vi "Main.vi"() -> ()   [LabVIEW 2015]
doc: "This template is for the Queued Message Handler design pattern.\n\nThe Event Handling Loop generates messages based on user interface actions.\n\nThe Message Handling Loop processes messages generated by the Event Handling Loop, or by other messages. The messages are string values, so new messages can be added easily to the Message Cases case structure in the Message Handling Loop. Each message cluster can also provide an optional value for Message Data, which is a variant that can be converted to whatever message-specific data is required."
uses:
  Controls & Type Defs/CurrentSong.ctl
  Controls & Type Defs/AlbumDetails.ctl
  Controls & Type Defs/UI Data.ctl
  Controls & Type Defs/AlbumArray.ctl
  Controls & Type Defs/ClickDetails.ctl
  Controls & Type Defs/SongTimerModes.ctl
  SubVIs/support/Message Queue/Enqueue Message (Single).vi
  <vilib>/Utility/error.llb/Error Cluster From Error Code.vi
  <vilib>/ErrorRing/Error Ring.xnode
  SubVIs/support/Message Queue/Message Queue.lvlib
  SubVIs/support/User Event - Stop/User Event - Stop.lvlib
panel:
  out "Album Details":T1={"Artist"="", "Album Name"="", "Songs"=-1}
  out "Current Song":T2
  in  "Pause":bool
  out "Playlist":i32(listbox)
  in  "Skip Forward":bool
  in  "Skip Back":bool
  in  "Media Stop Button":bool
  in  "Play":bool
  out "Time Remaining":dbl format="%<%M:%S>T"
  out "Song Progress":dbl(slide) scale=0.0..141.0 scale format="%<%M:%S>t"
  in  "Previous Album":bool
  in  "Next Album":bool
  out "Album Index":string
  out "Status":string
  in  "Exit":bool
  # "MP3 Player"
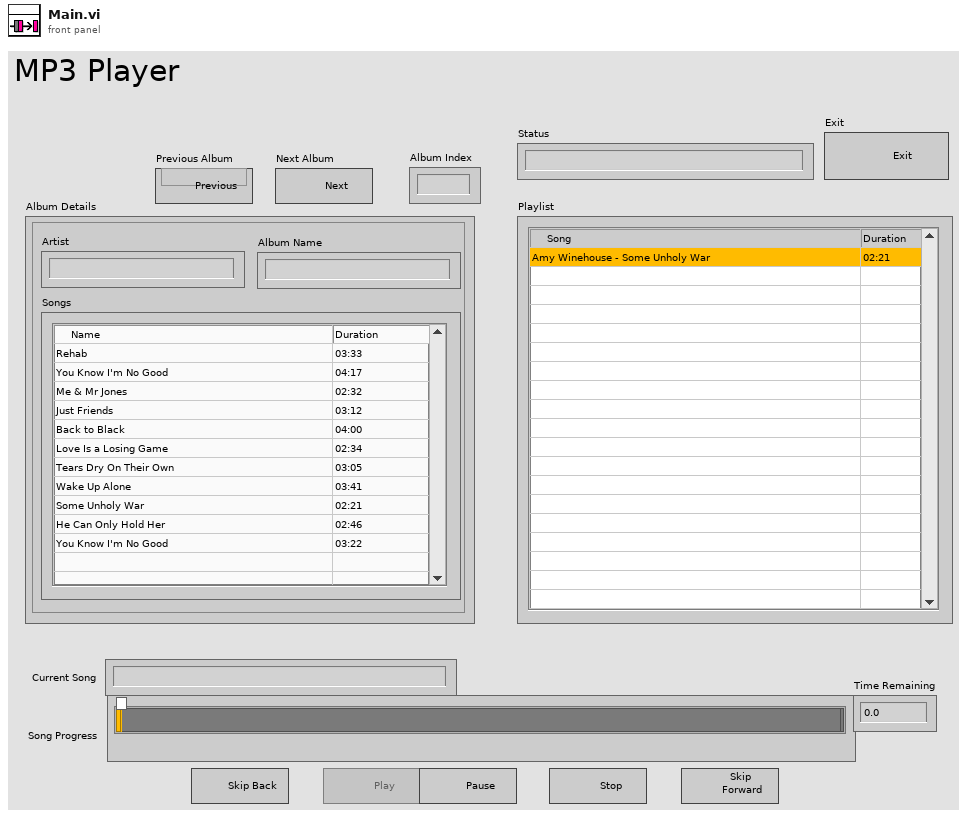
[diagram p1: front panel]
types:
  T1 = typedef "AlbumDetails.ctl" = cluster{"Artist":string, "Album Name":string, "Songs":i32}
  T2 = typedef "CurrentSong.ctl" = string
  T3 = typedef "AlbumArray.ctl" = cluster{"Artist Name":string, "Album Name":string, "Song Details":string[][]}[]
  T4 = typedef "UI Data.ctl" = cluster{"Album Index":refnum<vi>, "Album Details":refnum<vi>, "Add Button":refnum<vi>, "Remove Button":refnum<vi>, "Previous Album":refnum<vi>, "Next Album":refnum<vi>, "Song Progress":refnum<vi>, "Play":refnum<vi>, "Pause ":refnum<vi>, "Skip Forward":refnum<vi>, "Skip Back":refnum<vi>, "Media Stop Button":refnum<vi>, "Exit":refnum<vi>, "Playlist":refnum<vi>, "Current Song":refnum<vi>, "Time Remaining":refnum<vi>, "Status":refnum<vi>}
  T5 = typedef "Message Queue.lvlib/All Message Queues.ctl" = cluster{"UI":refnum<queue>, "Media":refnum<queue>}
  T6 = typedef "SongTimerModes.ctl" = enum16{"Start", "Play", "Jump"}
  T7 = typedef "ClickDetails.ctl" = cluster{"Coords":cluster{"Vertical":i32, "Horizontal":i32}, "MCLB Ref":refnum<vi>, "Button":u16}
  T8 = typedef "LVPoint32TypeDef.ctl" = cluster{"Horizontal":i32, "Vertical":i32}
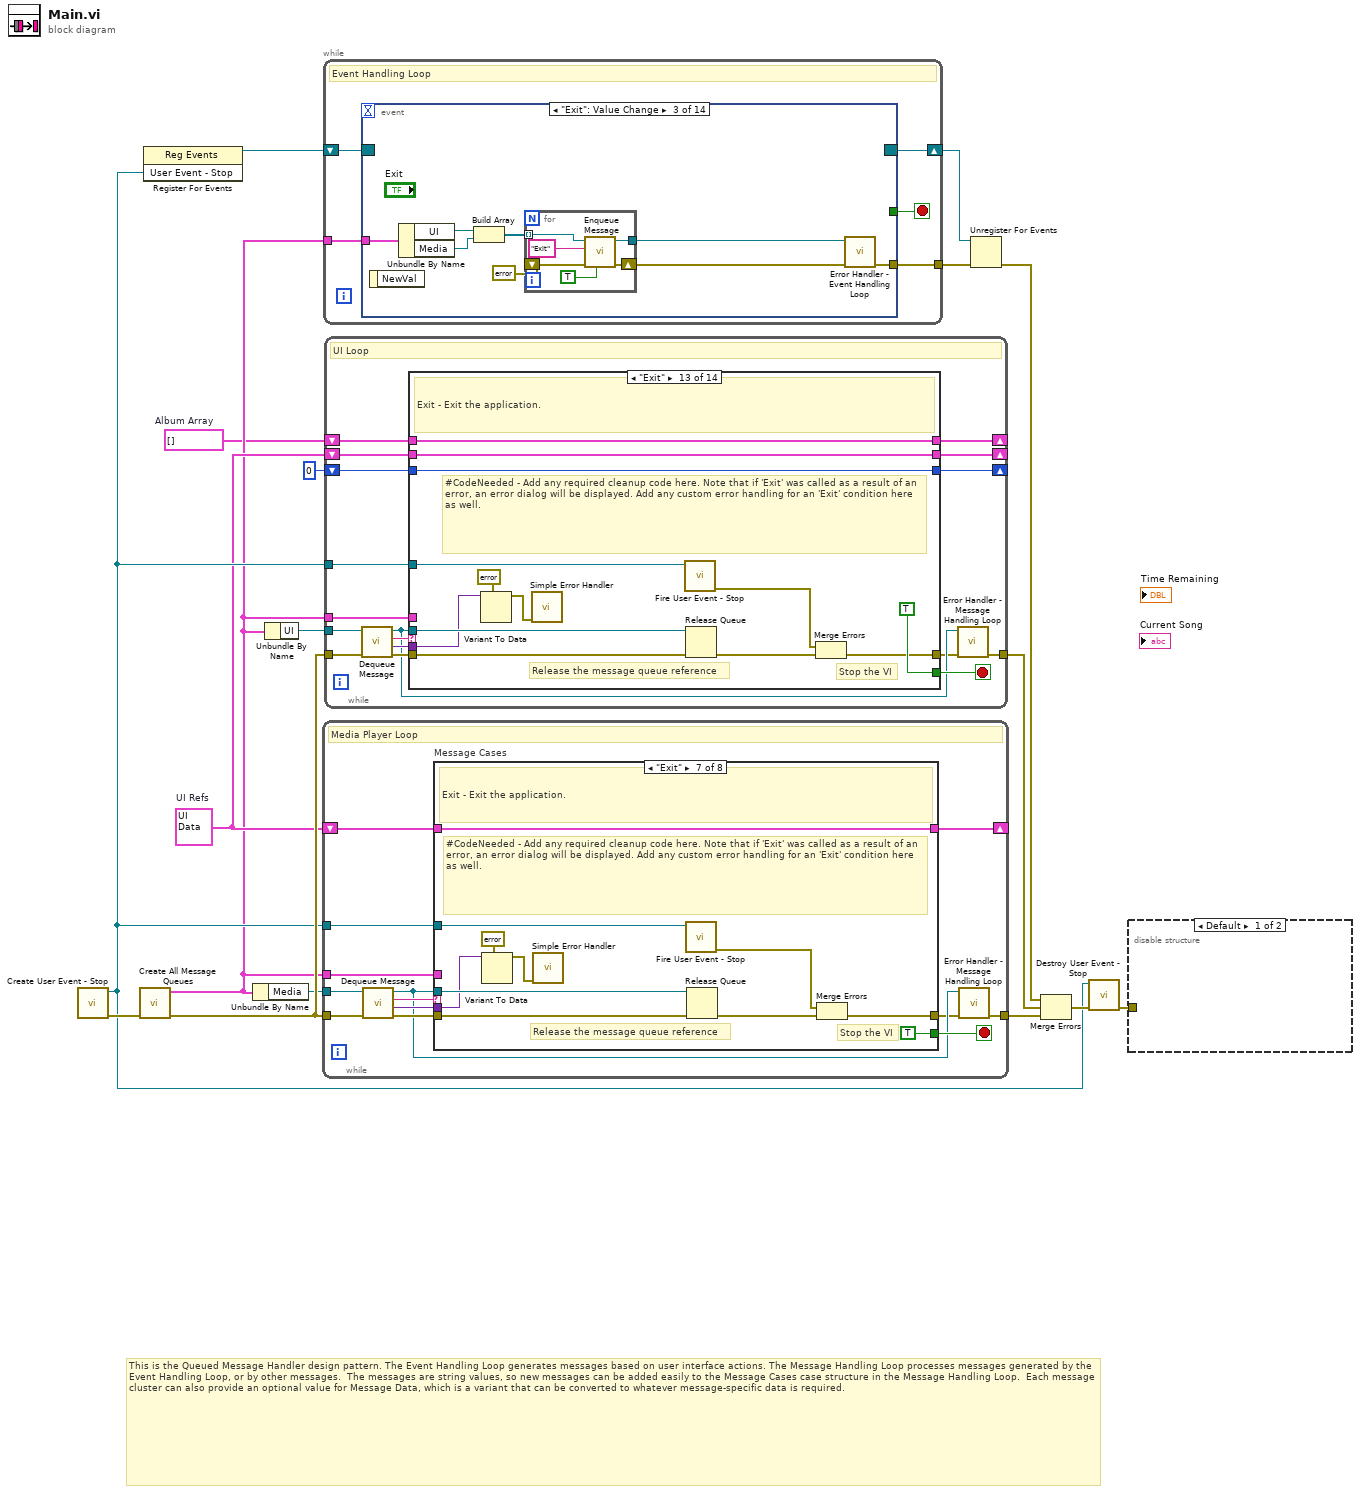
[diagram p0: block diagram]
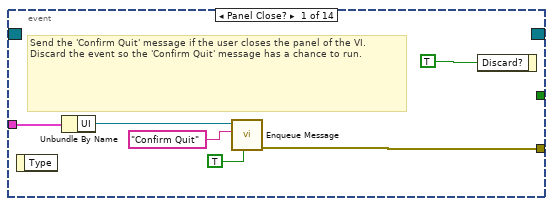
[diagram p2: hidden frame]
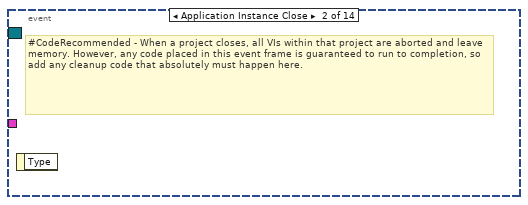
[diagram p3: hidden frame]
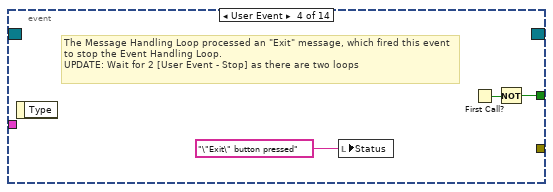
[diagram p4: hidden frame]
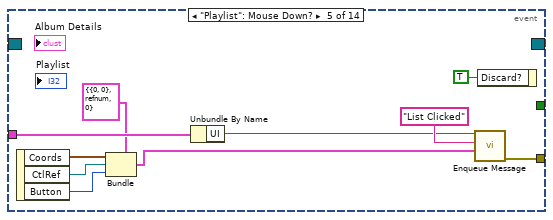
[diagram p5: hidden frame]
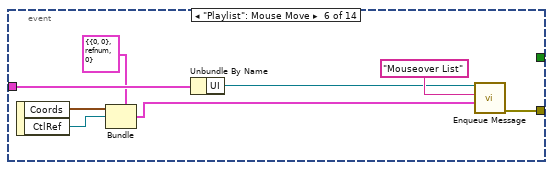
[diagram p6: hidden frame]
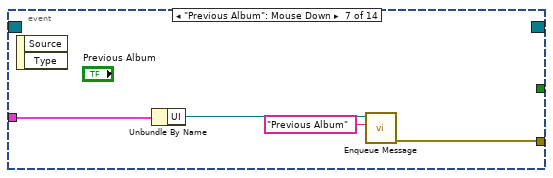
[diagram p7: hidden frame]
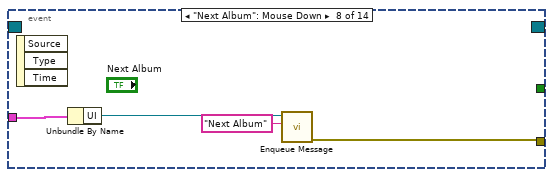
[diagram p8: hidden frame]
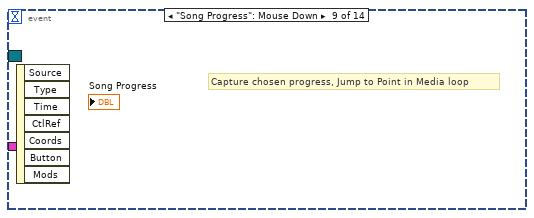
[diagram p9: hidden frame]
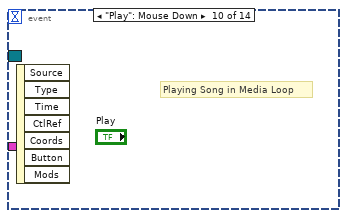
[diagram p10: hidden frame]
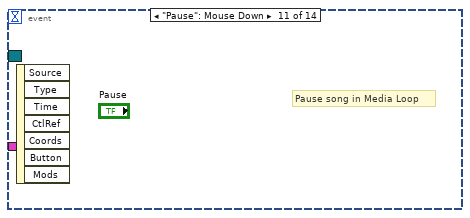
[diagram p11: hidden frame]
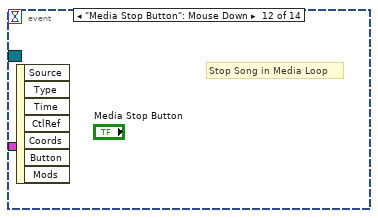
[diagram p12: hidden frame]
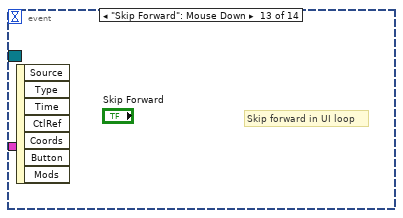
[diagram p13: hidden frame]
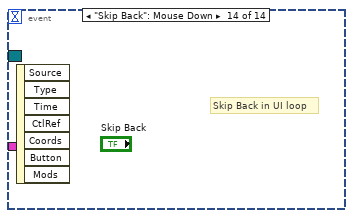
[diagram p14: hidden frame]
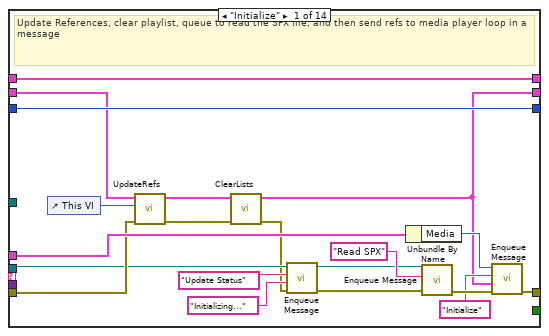
[diagram p15: hidden frame]
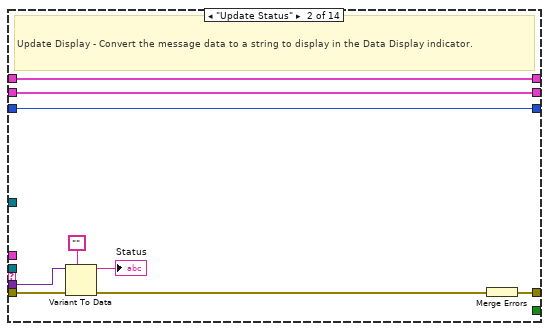
[diagram p16: hidden frame]
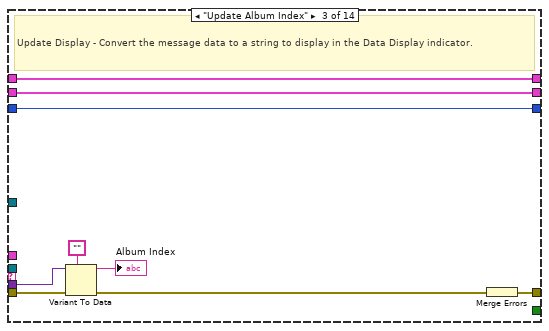
[diagram p17: hidden frame]
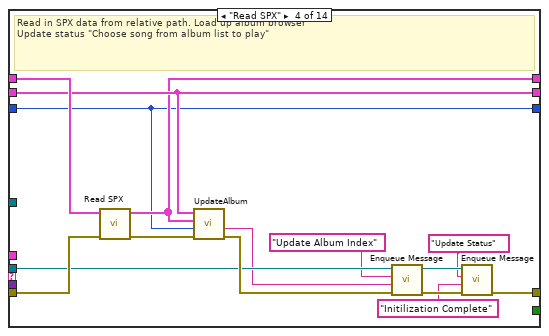
[diagram p18: hidden frame]
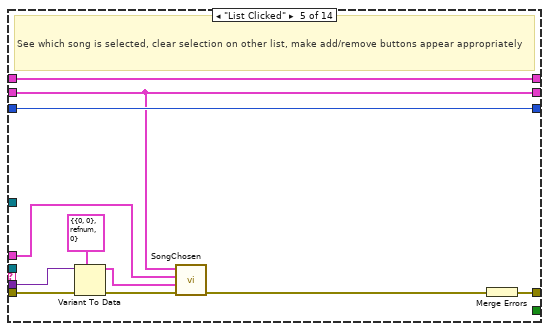
[diagram p19: hidden frame]
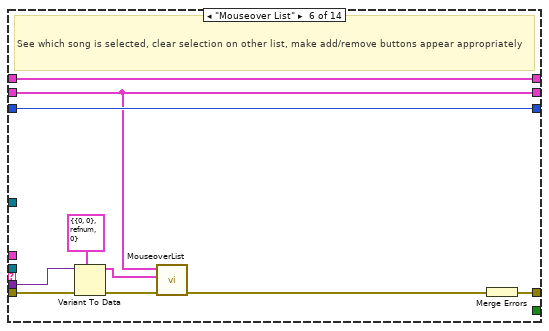
[diagram p20: hidden frame]
diagram:
  w1 = T3 []  # Album Array
  w8 = T4 {"Album Index"=refnum, "Album Details"=refnum, "Add Button"=refnum, "Remove Button"=refnum, "Previous Album"=refnum, "Next Album"=refnum, "Song Progress"=refnum, "Play"=refnum, "Pause "=refnum, "Skip Forward"=refnum, "Skip Back"=refnum, "Media Stop Button"=refnum, "Exit"=refnum, "Playlist"=refnum, "Current Song"=refnum, "Time Remaining"=refnum, "Status"=refnum}  # UI Refs
  # "This is the Queued Message Handler design pattern. The Event Handling Loop generates messages based on user interface actions. The Message Handling Loop processes messages generated by the Event Handling Loop, or by other messages.  The messages are string values, so new messages can be added easily to the Message Cases case structure in the Message Handling Loop.  Each message cluster can also provide an optional value for Message Data, which is a variant that can be converted to whatever message-specific data is required."
  n1 = call "Create User Event - Stop.vi"() -> ("error out"=w15:errorcluster, "User Event - Stop"=w9:refnum<user-event>)  [unwired: 10 in]
  n2 = call "Create All Message Queues.vi"("error in (no error)"=w15) -> ("error out"=w10:errorcluster, "Message Queues out"=w3:T5)  [unwired: 9 in]
  n3 = register-events(w9) -> (reference out=w11:refnum<event-registration>)  [unwired: 2 in, 1 out]
  n4 = Unbundle By Name(w3) -> ("Media"=w5:refnum<queue>)
  n5 = Unbundle By Name(w3) -> ("UI"=w4:refnum<queue>)
  n6 = while {
    tunnel: w5 -> [w22]
    shift-right: [w29] -> _
    shift-left: w8 -> [w30]
    tunnel: w9 -> [w27]
    tunnel: w10 -> [w26]
    tunnel: [w20] -> w16
    tunnel: w3 -> [w18]
    stop <- w28 stop-if-true
    # "Media Player Loop"
    n7 = call "Dequeue Message.vi"("error in (no error)"=w26, "Message Queue"=w22) -> ("error out"=w25:errorcluster, "Message Data"=w23:variant, "Message"=w24:string, "dup Message Queue"=w21:refnum<queue>)  [unwired: 6 in]
    n8 = case "Message Cases" shown="\"Exit\"" w24 {
      selector: w24 -> [_ _ _ _ _ _ _ w83]
      tunnel: w21 -> [_ _ w50 _ _ _ w81 _]
      tunnel: w25 -> [w35 w47 w56 w64 w67 w70 w74 _]
      tunnel: [w32 w49 w59 w62 w65 w68 w77 w84] -> w19
      tunnel: w30 -> [w36 w48 w57 w63 w66 w69 w80 w85]
      tunnel: [w31 w41 w55 w63 w66 w69 w80 w85] -> w29
      tunnel: [_ _ _ _ _ _ TRUE _] -> w28
      tunnel: w23 -> [w37 w46 _ _ _ _ w71 _]
      tunnel: w27 -> [_ _ _ _ _ _ w76 _]
      tunnel: w18 -> [_ w40 w58 _ _ _ _ _]
      frame "Initialize" {
        # "Read in previously loaded references from Browse & Playlist loop initilization case"
        n9 = Variant To Data(error in=w35, type=w36, Variant=w37) -> (data=w34:T4, error out=w33:errorcluster)
        n10 = call "ResetMedia.vi"("error in (no error)"=w33, "UI Refs"=w34) -> ("error out"=w32:errorcluster, "UI Refs"=w31:T4)  [unwired: 8 in]
      }
      frame "Start Song" {
        # "Ungrey Song Progress & other buttons, grey play button, update Current Song, update Status , Song Progress, Time remaining"
        n11 = call "StartSong.vi"("error in"=w47, "Message Data"=w46, "Message Queues"=w40, "UI Refs in"=w48) -> ("error out"=w45:errorcluster, "Message Queues"=w39:T5, "UI Refs out"=w44:T4, "Duration"=w43:dbl)  [unwired: 4 in]
        n12 = call "SongTimer.vi"("Time"=w43, "error in (no error)"=w45, "Mode"=SongTimerModes."Start", "Message Queues in"=w39, "UI Refs in"=w44) -> ("error out"=w38:errorcluster, "UI Refs out"=w41:T4)  [unwired: 5 in]
        n13 = Merge Errors(w38) -> (w49:errorcluster)
      }
      frame "Playing Song" {
        # "Update Song Progress, Current Song, Time Remaining, Check if song done, wait .1s"
        n14 = call "SongTimer.vi"("error in (no error)"=w56, "Message Queues in"=w58, "UI Refs in"=w57) -> ("error out"=w54:errorcluster, "UI Refs out"=w55:T4)  [unwired: 7 in]
        n15 = flat-sequence {
          tunnel: w54 -> [w60]
          tunnel: [w60] -> w53
          frame #0 {
            n16 = Wait (ms)(milliseconds to wait=u32 500) -> ()  [unwired: 1 out]
          }
        }
        n17 = call-poly "Enqueue Message.vi"("error in (no error)"=w53, "Message"="Playing Song", "Message Queue"=w50) -> ("error out"=w52:errorcluster)  [unwired: 7 in, 1 out]
        n18 = Merge Errors(w52) -> (w59:errorcluster)
      }
      frame "Jump to Point" {
        # "Convert % to seconds, set timer, update Song Progress, update time remaining"
        n19 = Merge Errors(w64) -> (w62:errorcluster)
      }
      frame "Pause Song" {
        # "Grey out Pause button, ungrey Play button"
        n20 = Merge Errors(w67) -> (w65:errorcluster)
      }
      frame "Stop Song" {
        # "Grey out Stop&Pause button, ungrey Play button"
        n21 = Merge Errors(w70) -> (w68:errorcluster)
      }
      frame "Exit" {
        # "Stop the VI"
        # "Release the message queue reference"
        # "#CodeNeeded - Add any required cleanup code here. Note that if 'Exit' was called as a result of an error, an error dialog will be displayed. Add any custom error handling for an 'Exit' condition here as well."
        # "Exit - Exit the application."
        n22 = Variant To Data(type=errorcluster {"status"=FALSE, "code"=0, "source"=""} ("error constant"), Variant=w71) -> (data=w72:errorcluster)  [unwired: 1 in, 1 out]
        n23 = call <vilib>:"Simple Error Handler.vi"("error in (no error)"=w72) -> ()  [unwired: 4 in, 5 out]
        n24 = call "Fire User Event - Stop.vi"("User Event - Stop"=w76) -> ("error out"=w75:errorcluster)  [unwired: 10 in]
        n25 = Release Queue(queue=w81, error in (no error)=w74) -> (error out=w78:errorcluster)  [unwired: 1 in, 2 out]
        n26 = Merge Errors(w75, w78) -> (w77:errorcluster)
      }
      frame Default {
        # "'Default' case only runs if there is a message that isn't defined in any of the other cases.  Output a programming error."
        n27 = xnode "Error Ring"("parameter 0"=w83) -> ("error out"=w84:errorcluster)
        n28 = One Button Dialog(message="Unknown command on Media Player Loop") -> ()  [unwired: 1 in, 1 out]
      }
    }
    n29 = call "Error Handler - Message Handling Loop.vi"("error in (no error)"=w19, "Message Queue"=w21) -> ("dup error in"=w20:errorcluster)  [unwired: 8 in, 1 out]
  }
  n30 = while {
    tunnel: w3 -> [w97]
    shift-right: [w95] -> w13
    shift-left: w11 -> [w96]
    tunnel: [w93] -> w12
    stop <- w94 stop-if-true
    # "Event Handling Loop"
    n31 = event shown="[2] \"Exit\": Value Change" {
      selector: w96 -> [_ _ _ _ _ _ _ _ _ _ _ _ _ _]
      dyn-events: [_ _ _ _ _ _ _ _ _ _ _ _ _ _] -> w95
      timeout: _ -> [_ _ _ _ _ _ _ _ _ _ _ _ _ _]
      tunnel: [_ _ _ w118 _ _ _ _ _ _ _ _ _ _] -> w94
      tunnel: w97 -> [w99 _ w108 _ w125 w133 w140 w146 _ _ _ _ _ _]
      tunnel: [w102 _ w109 _ w128 w136 w139 w143 _ _ _ _ _ _] -> w93
      event Panel Close? {
        # "Send the 'Confirm Quit' message if the user closes the panel of the VI. Discard the event so the 'Confirm Quit' message has a chance to run."
        n32 = event-data() -> ()  [unwired: 1 in, 1 out]
        n33 = Unbundle By Name(w99) -> ("UI"=w98:refnum<queue>)
        n34 = call-poly "Enqueue Message.vi"("Priority Message? (F)"=TRUE, "Message"="Confirm Quit", "Message Queue"=w98) -> ("error out"=w102:errorcluster)  [unwired: 7 in, 1 out]
        n35 = event-data("Discard?"=TRUE) -> ()  [unwired: 1 in, 1 out]
      }
      event Application Instance Close {
        # "#CodeRecommended - When a project closes, all VIs within that project are aborted and leave memory. However, any code placed in this event frame is guaranteed to run to completion, so add any cleanup code that absolutely must happen here."
        n36 = event-data() -> ()  [unwired: 1 in, 1 out]
      }
      event "Exit": Value Change {
        n37 = event-data() -> ()  [unwired: 1 in, 1 out]
        n38 = Unbundle By Name(w108) -> ("UI"=w107:refnum<queue>, "Media"=w106:refnum<queue>)
        n39 = Build Array(w107, w106) -> (w105:refnum<queue>[])
        n40 = for {
          tunnel: [w115] -> w111
          shift-right: [w114] -> w110
          shift-left: errorcluster {"status"=FALSE, "code"=0, "source"=""} ("error out") -> [w113]
          tunnel: w105 -> [w112] mode=indexing
          n41 = call-poly "Enqueue Message.vi"("Priority Message? (F)"=TRUE, "error in (no error)"=w113, "Message"="Exit", "Message Queue"=w112) -> ("error out"=w114:errorcluster, "dup Message Queue"=w115:refnum<queue>)  [unwired: 6 in]
        }
        n42 = call "Error Handler - Event Handling Loop.vi"("error in (no error)"=w110, "Message Queue"=w111) -> ("dup error in"=w109:errorcluster)  [unwired: 8 in, 1 out]
      }
      event User Event {
        # "The Message Handling Loop processed an \"Exit\" message, which fired this event to stop the Event Handling Loop. \nUPDATE: Wait for 2 [User Event - Stop] as there are two loops"
        n43 = event-data() -> ()  [unwired: 1 in, 1 out]
        n44 = local write "Status"("\"Exit\" button pressed" ("VI Stopped")) -> ()
        n45 = First Call?() -> (First Call?: T/F=w119:bool)
        n46 = Not(x=w119) -> (.not. x?=w118:bool)
      }
      event "Playlist": Mouse Down? {
        n47 = event-data() -> ("Coords"=w130:T8, "CtlRef"=w129:refnum<vi>, "Button"=w123:u16)  [unwired: 1 in]
        n48 = Bundle(cluster=T7 {"Coords"={"Vertical"=0, "Horizontal"=0}, "MCLB Ref"=refnum, "Button"=0} ("output cluster"), "Coords"=w130, "MCLB Ref"=w129, "Button"=w123) -> (w127:T7)
        n49 = Unbundle By Name(w125) -> ("UI"=w124:refnum<queue>)
        n50 = call-poly "Enqueue Message.vi"("Message Data"=w127, "Message"="List Clicked", "Message Queue"=w124) -> ("error out"=w128:errorcluster)  [unwired: 7 in, 1 out]
        n51 = event-data("Discard?"=TRUE) -> ()  [unwired: 1 in, 1 out]
      }
      event "Playlist": Mouse Move {
        n52 = event-data() -> ("Coords"=w138:T8, "CtlRef"=w137:refnum<vi>)  [unwired: 1 in]
        n53 = Bundle(cluster=T7 {"Coords"={"Vertical"=0, "Horizontal"=0}, "MCLB Ref"=refnum, "Button"=0} ("output cluster"), "Coords"=w138, "MCLB Ref"=w137) -> (w135:T7)  [unwired: 1 in]
        n54 = Unbundle By Name(w133) -> ("UI"=w132:refnum<queue>)
        n55 = call-poly "Enqueue Message.vi"("Message Data"=w135, "Message"="Mouseover List", "Message Queue"=w132) -> ("error out"=w136:errorcluster)  [unwired: 7 in, 1 out]
      }
      event "Previous Album": Mouse Down {
        n56 = event-data() -> ()  [unwired: 1 in, 2 out]
        n57 = Unbundle By Name(w140) -> ("UI"=w142:refnum<queue>)
        n58 = call-poly "Enqueue Message.vi"("Message"="Previous Album", "Message Queue"=w142) -> ("error out"=w139:errorcluster)  [unwired: 8 in, 1 out]
      }
      event "Next Album": Mouse Down {
        n59 = event-data() -> ()  [unwired: 1 in, 3 out]
        n60 = Unbundle By Name(w146) -> ("UI"=w145:refnum<queue>)
        n61 = call-poly "Enqueue Message.vi"("Message"="Next Album", "Message Queue"=w145) -> ("error out"=w143:errorcluster)  [unwired: 8 in, 1 out]
      }
      event "Song Progress": Mouse Down {
        # "Capture chosen progress, Jump to Point in Media loop"
        n62 = event-data() -> ()  [unwired: 1 in, 7 out]
      }
      event "Play": Mouse Down {
        # "Playing Song in Media Loop"
        n63 = event-data() -> ()  [unwired: 1 in, 7 out]
      }
      event "Pause": Mouse Down {
        # "Pause song in Media Loop"
        n64 = event-data() -> ()  [unwired: 1 in, 7 out]
      }
      event "Media Stop Button": Mouse Down {
        # "Stop Song in Media Loop"
        n65 = event-data() -> ()  [unwired: 1 in, 7 out]
      }
      event "Skip Forward": Mouse Down {
        # "Skip forward in UI loop"
        n66 = event-data() -> ()  [unwired: 1 in, 7 out]
      }
      event "Skip Back": Mouse Down {
        # "Skip Back in UI loop"
        n67 = event-data() -> ()  [unwired: 1 in, 7 out]
      }
    }
  }
  n68 = while {
    tunnel: w4 -> [w155]
    shift-right: [w162] -> _
    shift-left: w8 -> [w163]
    tunnel: w9 -> [w160]
    tunnel: w10 -> [w159]
    tunnel: [w153] -> w6
    shift-right: [w147] -> _
    shift-left: w1 -> [w151]
    tunnel: w3 -> [w150]
    shift-right: [w148] -> _
    shift-left: 0 -> [w149]
    stop <- w161 stop-if-true
    # "UI Loop"
    n69 = call "Dequeue Message.vi"("error in (no error)"=w159, "Message Queue"=w155) -> ("error out"=w158:errorcluster, "Message Data"=w156:variant, "Message"=w157:string, "dup Message Queue"=w154:refnum<queue>)  [unwired: 6 in]
    n70 = case "Message Cases" shown="\"Exit\"" w157 {
      selector: w157 -> [_ _ _ _ _ _ _ _ _ _ _ _ _ w312]
      tunnel: w154 -> [w171 _ _ w209 _ _ w240 w258 _ _ _ w291 w308 _]
      tunnel: w158 -> [w174 w190 w199 w216 w223 w233 w244 w262 w272 w277 w286 w295 w301 _]
      tunnel: [w181 w191 w200 w204 w227 w237 w242 w260 w270 w275 w280 w293 w304 w313] -> w152
      tunnel: w163 -> [w173 w192 w201 w214 w221 w231 w247 w264 w271 w276 w285 w294 w307 w314]
      tunnel: [w167 w192 w201 w214 w221 w231 w247 w264 w271 w276 w285 w294 w307 w314] -> w162
      tunnel: [_ _ _ _ _ _ _ _ _ _ _ _ TRUE _] -> w161
      tunnel: w156 -> [_ w189 w198 _ w224 w234 _ _ _ _ w284 _ w298 _]
      tunnel: w160 -> [_ _ _ _ _ _ _ _ _ _ _ _ w303 _]
      tunnel: w151 -> [w176 w184 w194 w215 w225 w235 w246 w263 w268 w273 w278 w287 w296 w309]
      tunnel: [w176 w184 w194 w212 w225 w235 w246 w263 w268 w273 w278 w287 w296 w309] -> w147
      tunnel: w150 -> [w182 _ _ _ w217 _ _ _ _ _ _ _ _ _]
      tunnel: w149 -> [w177 w185 w195 w211 w226 w236 w245 w254 w269 w274 w279 w288 w297 w310]
      tunnel: [w177 w185 w195 w211 w226 w236 w243 w261 w269 w274 w279 w288 w297 w310] -> w148
      frame "Initialize" {
        # "Update References, clear playlist, queue to read the SPX file, and then send refs to media player loop in a message"
        n71 = control-ref of="This VI"() -> (w175:refnum<vi>)
        n72 = call "UpdateRefs.vi"("Error In"=w174, "VI Ref In"=w175, "UI Refs in"=w173) -> ("Error Out"=w165:errorcluster, "UI Refs out"=w172:T4)  [unwired: 7 in]
        n73 = call "ClearLists.vi"("error in (no error)"=w165, "UI Refs"=w172) -> ("error out"=w166:errorcluster, "UI Refs"=w167:T4)  [unwired: 8 in]
        n74 = call-poly "Enqueue Message.vi"("error in (no error)"=w166, "Message Data"="Initializing..." ("Message"), "Message"="Update Status", "Message Queue"=w171) -> ("error out"=w164:errorcluster, "dup Message Queue"=w170:refnum<queue>)  [unwired: 6 in]
        n75 = Unbundle By Name(w182) -> ("Media"=w179:refnum<queue>)
        n76 = call-poly "Enqueue Message.vi"("error in (no error)"=w164, "Message"="Read SPX", "Message Queue"=w170) -> ("error out"=w180:errorcluster)  [unwired: 7 in, 1 out]
        n77 = call-poly "Enqueue Message.vi"("error in (no error)"=w180, "Message Data"=w167, "Message"="Initialize", "Message Queue"=w179) -> ("error out"=w181:errorcluster)  [unwired: 6 in, 1 out]
      }
      frame "Update Status" {
        # "Update Display - Convert the message data to a string to display in the Data Display indicator."
        n78 = Variant To Data(error in=w190, type="", Variant=w189) -> (data=→"Status":string, error out=w187:errorcluster)
        n79 = Merge Errors(w187) -> (w191:errorcluster)
      }
      frame "Update Album Index" {
        # "Update Display - Convert the message data to a string to display in the Data Display indicator."
        n80 = Variant To Data(error in=w199, type="", Variant=w198) -> (data=→"Album Index":string, error out=w196:errorcluster)
        n81 = Merge Errors(w196) -> (w200:errorcluster)
      }
      frame "Read SPX" {
        # "Read in SPX data from relative path. Load up album browser\nUpdate status \"Choose song from album list to play\""
        n82 = call "Read SPX.vi"("error in (no error)"=w216, "All Albums"=w215) -> ("error out"=w213:errorcluster, "All Albums"=w212:T3)  [unwired: 8 in]
        n83 = call "UpdateAlbum.vi"("error in"=w213, "Album Index"=w211, "AlbumArray"=w212, "UI Refs"=w214) -> ("error out"=w210:errorcluster, "Album Index"=w207:string)  [unwired: 6 in]
        n84 = call-poly "Enqueue Message.vi"("error in (no error)"=w210, "Message Data"=w207, "Message"="Update Album Index", "Message Queue"=w209) -> ("error out"=w205:errorcluster, "dup Message Queue"=w206:refnum<queue>)  [unwired: 6 in]
        n85 = call-poly "Enqueue Message.vi"("error in (no error)"=w205, "Message Data"="Initilization Complete" ("Message"), "Message"="Update Status", "Message Queue"=w206) -> ("error out"=w204:errorcluster)  [unwired: 6 in, 1 out]
      }
      frame "List Clicked" {
        # "See which song is selected, clear selection on other list, make add/remove buttons appear appropriately"
        n86 = Variant To Data(error in=w223, type=T7 {"Coords"={"Vertical"=0, "Horizontal"=0}, "MCLB Ref"=refnum, "Button"=0} ("output cluster"), Variant=w224) -> (data=w218:T7, error out=w220:errorcluster)
        n87 = call "SongChosen.vi"("error in (no error)"=w220, "Click Details"=w218, "Message Queues"=w217, "UI Refs"=w221) -> ("error out"=w219:errorcluster)  [unwired: 7 in]
        n88 = Merge Errors(w219) -> (w227:errorcluster)
      }
      frame "Mouseover List" {
        # "See which song is selected, clear selection on other list, make add/remove buttons appear appropriately"
        n89 = Variant To Data(error in=w233, type=T7 {"Coords"={"Vertical"=0, "Horizontal"=0}, "MCLB Ref"=refnum, "Button"=0} ("output cluster"), Variant=w234) -> (data=w228:T7, error out=w230:errorcluster)
        n90 = call "MouseoverList.vi"("error in (no error)"=w230, "Click Details"=w228, "UI Refs"=w231) -> ("error out"=w229:errorcluster)  [unwired: 8 in]
        n91 = Merge Errors(w229) -> (w237:errorcluster)
      }
      frame "Next Album" {
        # "Check if album index needs to roll over"
        # "Increment album index, check for rollover, index new album details, deselect any selections in list"
        n92 = Array Size(array=w246) -> (size(s)=w248:i32)
        n93 = Decrement(x=w248) -> (x-1=w249:i32)
        n94 = Equal?(x=w245, y=w249) -> (x = y?=w250:bool)
        n95 = Increment(x=w245) -> (x+1=w251:i32)
        n96 = Select(t=0, s=w250, f=w251) -> (s? t:f=w243:i32)
        n97 = call "UpdateAlbum.vi"("error in"=w244, "Album Index"=w243, "AlbumArray"=w246, "UI Refs"=w247) -> ("error out"=w241:errorcluster, "Album Index"=w239:string)  [unwired: 6 in]
        n98 = call-poly "Enqueue Message.vi"("error in (no error)"=w241, "Message Data"=w239, "Message"="Update Album Index", "Message Queue"=w240) -> ("error out"=w242:errorcluster)  [unwired: 6 in, 1 out]
      }
      frame "Previous Album" {
        # "Check if album index needs to roll over"
        # "Increment album index, check for rollover, index new album details, deselect any selections in list"
        n99 = Array Size(array=w263) -> (size(s)=w265:i32)
        n100 = Decrement(x=w265) -> (x-1=w253:i32)
        n101 = Equal?(x=0 ("t"), y=w254) -> (x = y?=w266:bool)
        n102 = Decrement(x=w254) -> (x-1=w267:i32)
        n103 = Select(t=w253, s=w266, f=w267) -> (s? t:f=w261:i32)
        n104 = call "UpdateAlbum.vi"("error in"=w262, "Album Index"=w261, "AlbumArray"=w263, "UI Refs"=w264) -> ("error out"=w259:errorcluster, "Album Index"=w257:string)  [unwired: 6 in]
        n105 = call-poly "Enqueue Message.vi"("error in (no error)"=w259, "Message Data"=w257, "Message"="Update Album Index", "Message Queue"=w258) -> ("error out"=w260:errorcluster)  [unwired: 6 in, 1 out]
      }
      frame "Skip Forward" {
        # "Remove Song in UI Loop. If playlist len=1, then Stop in Media Loop. If not, Start Song in Media Loop"
        n106 = Merge Errors(w272) -> (w270:errorcluster)
      }
      frame "Skip Back" {
        # "Stop then Play in Media Loop. If history queue created, then redevelop this code"
        n107 = Merge Errors(w277) -> (w275:errorcluster)
      }
      frame "Error" {
        # "#CodeRecommended - If you ever change the name of this \"Error\" message, you'll need to update the name in the Check Loop Error.vi as well."
        # "#CodeRecommended - Consider creating a system for logging errors in some way. These errors are for notification purposes only. Handling of specific errors should be performed in the message frames that generated the error."
        # "Error - Display an error dialog. This message is sent by the \"Error Handler\" VIs at the end of other loops in this application."
        n108 = Variant To Data(error in=w286, type=errorcluster {"status"=FALSE, "code"=0, "source"=""} ("error constant"), Variant=w284) -> (data=w282:errorcluster, error out=w281:errorcluster)
        n109 = call <vilib>:"Simple Error Handler.vi"("error in (no error)"=w282) -> ()  [unwired: 4 in, 5 out]
        n110 = Merge Errors(w281) -> (w280:errorcluster)
      }
      frame "Confirm Quit" {
        # "#CodeNeeded - If you want to provide an \"Are you sure\" dialog (or some other notification) before the application exits, place that code here. This message is typically sent from a Panel Close? event."
        # "Confirm Quit - Message that can confirm whether or not the user wants to exit the application."
        n111 = call-poly "Enqueue Message.vi"("Priority Message? (F)"=TRUE, "error in (no error)"=w295, "Message"="Exit", "Message Queue"=w291) -> ("error out"=w292:errorcluster)  [unwired: 6 in, 1 out]
        n112 = Merge Errors(w292) -> (w293:errorcluster)
      }
      frame "Exit" {
        # "Stop the VI"
        # "Release the message queue reference"
        # "#CodeNeeded - Add any required cleanup code here. Note that if 'Exit' was called as a result of an error, an error dialog will be displayed. Add any custom error handling for an 'Exit' condition here as well."
        # "Exit - Exit the application."
        n113 = Variant To Data(type=errorcluster {"status"=FALSE, "code"=0, "source"=""} ("error constant"), Variant=w298) -> (data=w299:errorcluster)  [unwired: 1 in, 1 out]
        n114 = call <vilib>:"Simple Error Handler.vi"("error in (no error)"=w299) -> ()  [unwired: 4 in, 5 out]
        n115 = call "Fire User Event - Stop.vi"("User Event - Stop"=w303) -> ("error out"=w302:errorcluster)  [unwired: 10 in]
        n116 = Release Queue(queue=w308, error in (no error)=w301) -> (error out=w305:errorcluster)  [unwired: 1 in, 2 out]
        n117 = Merge Errors(w302, w305) -> (w304:errorcluster)
      }
      frame Default {
        # "'Default' case only runs if there is a message that isn't defined in any of the other cases.  Output a programming error."
        n118 = xnode "Error Ring"("parameter 0"=w312) -> ("error out"=w313:errorcluster)
        n119 = One Button Dialog(message="Unknown command on Browse & Playlist Loop") -> ()  [unwired: 1 in, 1 out]
      }
    }
    n120 = call "Error Handler - Message Handling Loop.vi"("error in (no error)"=w152, "Message Queue"=w154) -> ("dup error in"=w153:errorcluster)  [unwired: 8 in, 1 out]
  }
  n121 = Unregister For Events(event registration refnum=w13, error in=w12) -> (error out=w7:errorcluster)
  n122 = Merge Errors(w7, w6, w16) -> (w14:errorcluster)
  n123 = call "Destroy User Event - Stop.vi"("error in (no error)"=w14, "User Event - Stop"=w9) -> ("error out"=w17:errorcluster)  [unwired: 9 in]
  n124 = disable-structure shown="Default" {
    disable-tunnel: w17 -> [_ _]
    frame condition #0 (active) {
    }
    frame condition #1 {
      # "Call Quit LabVIEW if running as a built application."
      n125 = Quit LabVIEW() -> ()  [unwired: 1 in]
    }
  }
